vi "CreateTrigImg.vi"(4 "Y Pixels":i32, 5 "Max Green":u16=65535, 6 "X Pixels":i32, 7 "Max Red":u16=65535, 8 "error in (no error)":errorcluster, 9 "Images In":T1[](array[typedef]), 10 "Green Data":u16[](array[numeric]), 11 "Red Data":u16[](array[numeric])) -> (0 "error out":errorcluster, 1 "Trig Img Out":T1, 2 "Red Image Out":T1, 3 "Green Image Out":T1)   [LabVIEW 2015]
uses:
  <vilib>/vision/Image Controls.llb/IMAQ Image.ctl
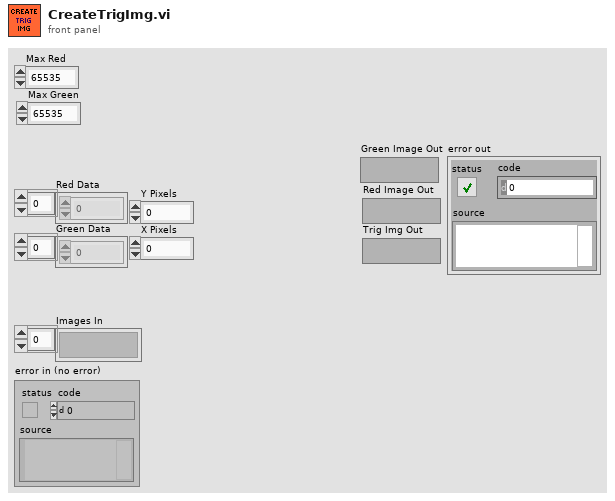
[diagram p1: front panel]
types:
  T1 = typedef "IMAQ Image.ctl" = refnum<image>
  T2 = cluster{"element":u16, "element":u16, u16, "n":u16}[][]
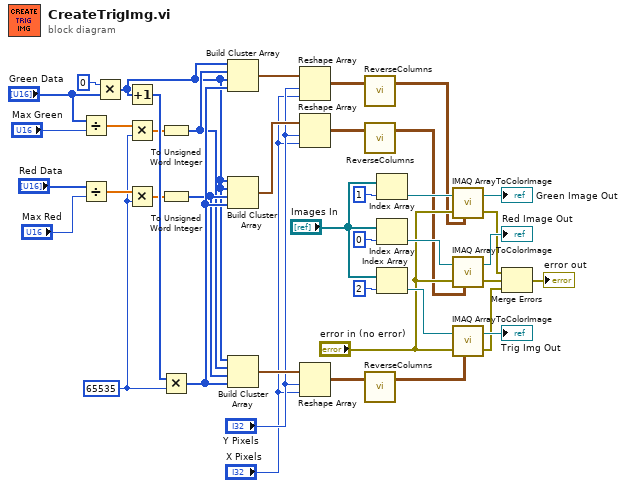
[diagram p0: block diagram]
diagram:
  w21 = u16 65535
  n1 = Divide(x="Green Data", y="Max Green") -> (x/y=w26:dbl[])
  n2 = Divide(x="Red Data", y="Max Red") -> (x/y=w24:dbl[])
  n3 = Multiply(x=u16 0 ("element"), y="Green Data") -> (x*y=w17:u16[])
  n4 = Increment(x=w17) -> (x+1=w40:u16[])
  n5 = Multiply(x=w26, y=w21) -> (x*y=w27:dbl[])
  n6 = Multiply(x=w24, y=w21) -> (x*y=w25:dbl[])
  n7 = To Unsigned Word Integer(number=w27) -> (unsigned 16bit integer=w22:u16[])
  n8 = To Unsigned Word Integer(number=w25) -> (unsigned 16bit integer=w23:u16[])
  n9 = Multiply(x=w40, y=w21) -> (x*y=w39:u16[])
  n10 = Build Cluster Array(w17, w22, w17, w39) -> (w35:cluster{u16, u16, u16, u16}[])
  n11 = Build Cluster Array(w17, w17, w23, w39) -> (w38:cluster{u16, u16, u16, u16}[])
  n12 = Build Cluster Array(w17, w22, w23, w39) -> (w41:cluster{u16, u16, u16, u16}[])
  n13 = Reshape Array(w35, "Y Pixels", "X Pixels") -> (w2:cluster{u16, u16, u16, u16}[][])
  n14 = Reshape Array(w38, "Y Pixels", "X Pixels") -> (w4:cluster{u16, u16, u16, u16}[][])
  n15 = Reshape Array(w41, "Y Pixels", "X Pixels") -> (w6:cluster{u16, u16, u16, u16}[][])
  n16 = call "ReverseColumns.vi"("output array 2"=w2) -> ("transposed array"=w1:T2)  [unwired: 2 in]
  n17 = call "ReverseColumns.vi"("output array 2"=w4) -> ("transposed array"=w3:T2)  [unwired: 2 in]
  n18 = call "ReverseColumns.vi"("output array 2"=w6) -> ("transposed array"=w5:T2)  [unwired: 2 in]
  n19 = Index Array(array="Images In", index=1) -> (element=w33:T1)
  n20 = Index Array(array="Images In", index=0) -> (element=w36:T1)
  n21 = Index Array(array="Images In", index=2) -> (element=w31:T1)
  n22 = call "IMAQ ArrayToColorImage"("Image"=w33, "Image Pixels (U64)"=w1, "error in (no error)"="error in (no error)") -> ("Image Out"=→"Green Image Out":T1, "error out"=w12:errorcluster)  [unwired: 2 in]
  n23 = call "IMAQ ArrayToColorImage"("Image"=w36, "Image Pixels (U64)"=w3, "error in (no error)"="error in (no error)") -> ("Image Out"=→"Red Image Out":T1, "error out"=w11:errorcluster)  [unwired: 2 in]
  n24 = call "IMAQ ArrayToColorImage"("Image"=w31, "Image Pixels (U64)"=w5, "error in (no error)"="error in (no error)") -> ("Image Out"=→"Trig Img Out":T1, "error out"=w10:errorcluster)  [unwired: 2 in]
  n25 = Merge Errors(w12, w11, w10) -> (→"error out":errorcluster)
